vi "TimeTasker.vi"(2 "Delay(sec)":dbl, 3 "Start Counting?":bool=TRUE, 4 "TeleOp Elapsed Seconds":dbl) -> (0 "Counting?":bool, 1 "TimePast?":bool)   [LabVIEW 2011]
uses:
  <vilib>/functionblocks/FB Core/FB Core.xnode
panel:
  out "elapsed time (ms)":i32
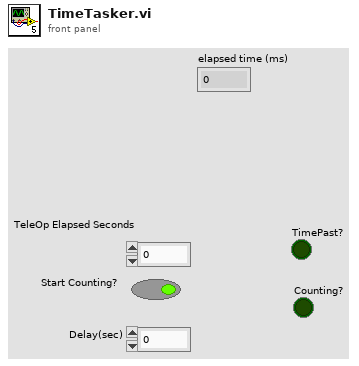
[diagram p1: front panel]
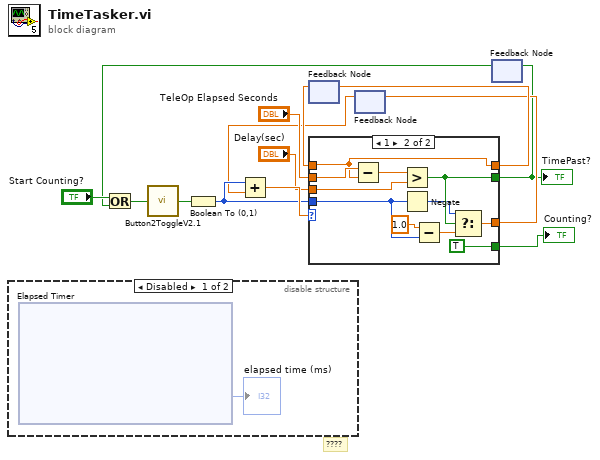
[diagram p0: block diagram]
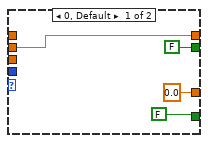
[diagram p2: hidden frame]
diagram:
  # "????"
  n1 = disable-structure shown="Disabled" {
    frame Disabled {
      n2 = xnode "Elapsed Timer"() -> ("elapsed time (ms)"=→"elapsed time (ms)":i32)  [unwired: 3 in, 1 out]
    }
    frame Enabled {
    }
  }
  n3 = feedback #1() -> (w11:dbl)  [unwired: 1 in]
  n4 = feedback #2() -> (w7:dbl)  [unwired: 1 in]
  n5 = feedback #3() -> (w3:bool)  [unwired: 1 in]
  n6 = Or(x="Start Counting?", y=w3) -> (x .or. y?=w6:bool)
  n7 = call "Button2ToggleV2.1.vi"("a"=w6) -> ("Result(clone)"=w5:bool)
  n8 = Boolean To (0,1)(Boolean=w5) -> (0, 1=w9:i16)
  n9 = Add(x=w9, y=w7) -> (x+y=w14:dbl)
  n10 = case shown="1" w14 {
    tunnel: [w19 w21] -> w12
    tunnel: "TeleOp Elapsed Seconds" -> [w19 w30]
    tunnel: w11 -> [_ w21]
    tunnel: [FALSE ("Start Counting?") w27] -> w2
    tunnel: "Delay(sec)" -> [_ w28]
    tunnel: w9 -> [_ w23]
    tunnel: [0.0 ("f") w25] -> w8
    tunnel: [FALSE ("Counting?") TRUE ("Counting?")] -> w1
    frame 0, Default {
    }
    frame 1 {
      n11 = Subtract(x=w30, y=w21) -> (x-y=w29:dbl)
      n12 = Greater?(x=w29, y=w28) -> (0:w27:bool)
      n13 = Negate(x=w23) -> (-x=w26:i16)
      n14 = Subtract(x=1.0 ("f"), y=w23) -> (x-y=w22:dbl)
      n15 = Select(t=w26, s=w27, f=w22) -> (s? t:f=w25:dbl)
    }
  }
  "TimePast?" <- w2
  "Counting?" <- w1
  n16 = feedback-in #1(w12) -> ()
  n17 = feedback-in #2(w8) -> ()
  n18 = feedback-in #3(w2) -> ()
